vi "StateHopper.vi"(0 "Master State In":T1(ring)) -> ()   [LabVIEW 2020]
doc: "This VI makes all decisions related to the hopper subsystem."
uses:
  <vilib>/Rock Robotics/WPI/DriverStation/WPI_DriverStationAllianceInfo.ctl
  635383ba-0535-4eb4-9430-5d5cc08842cb.vi
  GlobalDriverStationCommands.vi
  GlobalHopper.vi
  GlobalDriverStationData.vi
  GlobalGripper.vi
panel:
  in  "Delay for arm clearing (ms)":u32=800
  in  "Delay for wing retraction (ms)":u32=200
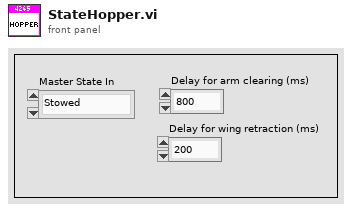
[diagram p1: front panel]
types:
  T1 = enum16{"Stowed", "Balancing", "Scoring", "Hoppering", "Ground", "Shelf"}
  T2 = typedef "WPI_DriverStationAllianceInfo.ctl" = enum16{"Red", "Blue", "Invalid"}
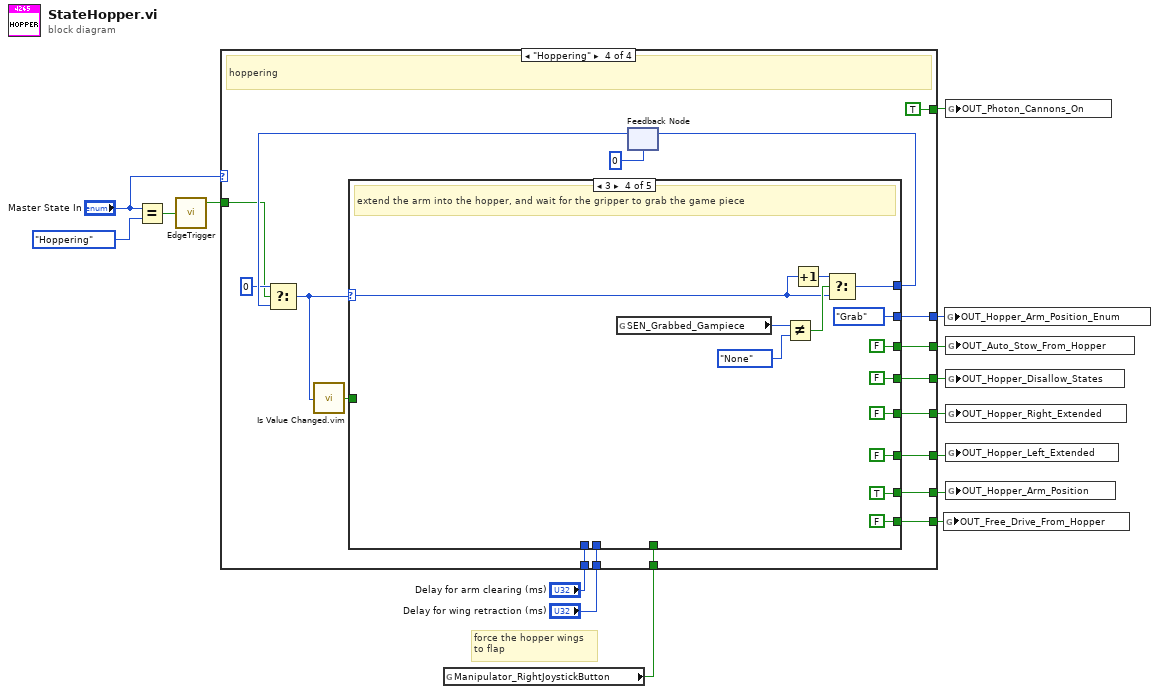
[diagram p0: block diagram]
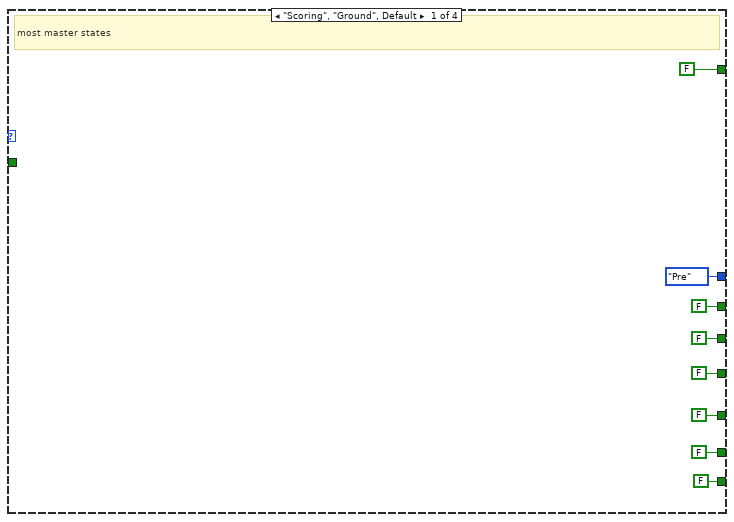
[diagram p2: hidden frame]
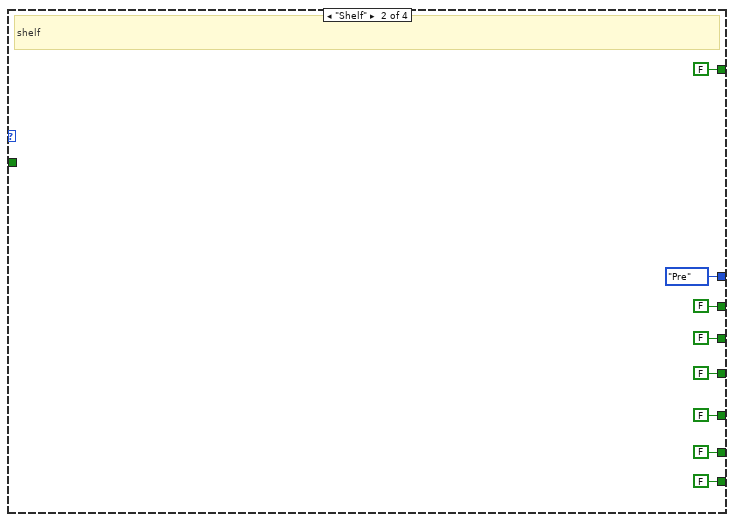
[diagram p3: hidden frame]
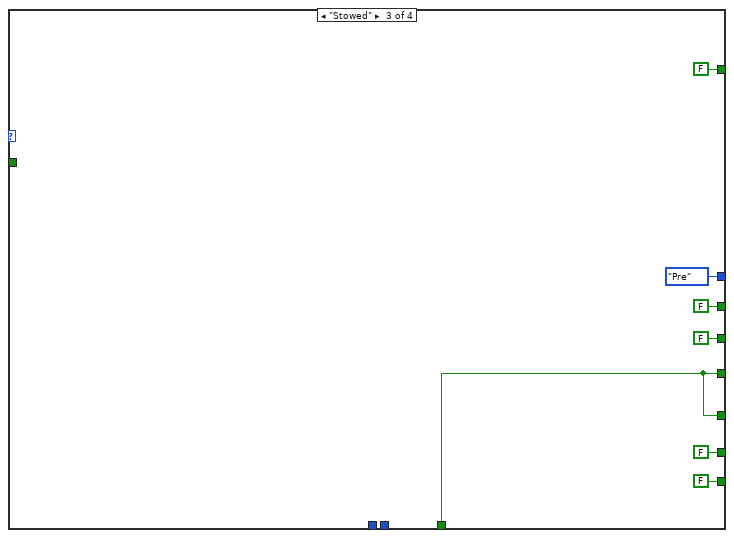
[diagram p4: hidden frame]
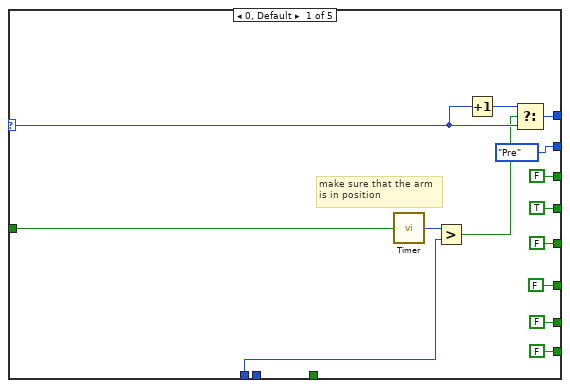
[diagram p5: hidden frame]
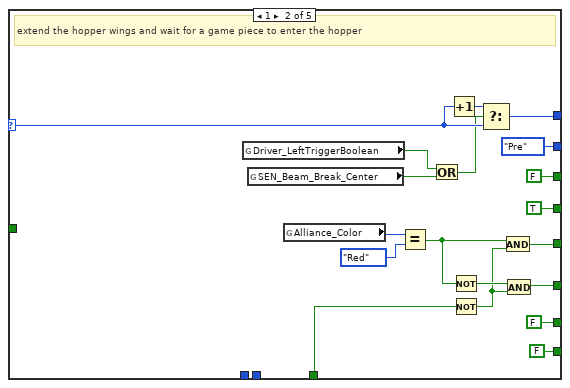
[diagram p6: hidden frame]
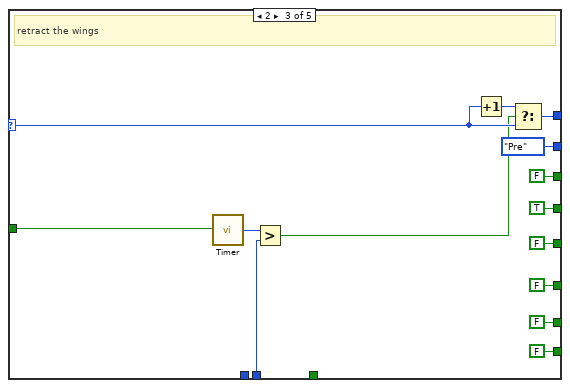
[diagram p7: hidden frame]
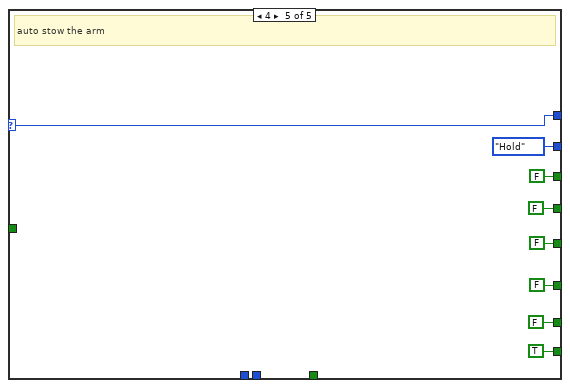
[diagram p8: hidden frame]
diagram:
  # "force the hopper wings\nto flap"
  n1 = Equal?(x="Master State In", y=T1."Hoppering") -> (x = y?=w9:bool)
  n2 = call "EdgeTrigger.vi"("Input Signal"=w9) -> ("Rising Edge Trigger"=w14:bool)  [unwired: 2 out]
  n3 = global read "GlobalDriverStationCommands.vi" "Manipulator_RightJoystickButton"() -> (w4:bool)
  n4 = case shown="\"Hoppering\"" "Master State In" {
    tunnel: w14 -> [_ _ _ w52]
    tunnel: [FALSE ("changed or first call?") FALSE ("changed or first call?") FALSE ("changed or first call?") w49] -> w13
    tunnel: [FALSE ("OUT_Hopper_Arm_Position") FALSE ("OUT_Hopper_Arm_Position") FALSE ("OUT_Hopper_Arm_Position") w48] -> w12
    tunnel: [FALSE ("OUT_Hopper_Arm_Position") FALSE ("OUT_Hopper_Arm_Position") FALSE ("OUT_Hopper_Arm_Position") w47] -> w11
    tunnel: [FALSE ("OUT_Hopper_Extended") FALSE ("New State") w35 w46] -> w10
    tunnel: "Delay for wing retraction (ms)" -> [_ _ _ w45]
    tunnel: [FALSE ("New State") FALSE ("New State") w35 w44] -> w7
    tunnel: [FALSE FALSE FALSE TRUE] -> w5
    tunnel: w4 -> [_ _ w35 w42]
    tunnel: "Delay for arm clearing (ms)" -> [_ _ _ w41]
    tunnel: [FALSE FALSE FALSE w40] -> w2
    tunnel: [enum16{"Pre", "Grab", "Hold"}."Pre" ("OUT_Hopper_Arm_Position_Enum") enum16{"Pre", "Grab", "Hold"}."Pre" ("OUT_Hopper_Arm_Position_Enum") enum16{"Pre", "Grab", "Hold"}."Pre" ("OUT_Hopper_Arm_Position_Enum") w39] -> w1
    frame "Scoring", "Ground", Default {
      # "most master states"
    }
    frame "Shelf" {
      # "shelf"
    }
    frame "Stowed" {
    }
    frame "Hoppering" {
      # "hoppering"
      n5 = feedback #1(0) -> (w54:i32)
      n6 = Select(t=0, s=w52, f=w54) -> (s? t:f=w50:i32)
      n7 = call "Is Value Changed.vim"("value"=w50) -> ("changed or first call?"=w51:bool)
      n8 = case shown="3" w50 {
        selector: w50 -> [w69 w87 w97 w113 w124]
        tunnel: [FALSE ("New State") w78 FALSE ("New State") FALSE ("Manipulator_RightJoystickButton") FALSE ("Manipulator_RightJoystickButton")] -> w46
        tunnel: [w70 w89 w99 w114 w124] -> w56
        tunnel: w51 -> [w60 _ w96 _ _]
        tunnel: [TRUE ("OUT_Hopper_Arm_Position") TRUE ("OUT_Hopper_Arm_Position") TRUE ("OUT_Hopper_Arm_Position") FALSE ("OUT_Hopper_Arm_Position") FALSE ("OUT_Hopper_Arm_Position")] -> w47
        tunnel: [FALSE ("OUT_Hopper_Arm_Position") FALSE ("OUT_Hopper_Arm_Position") FALSE ("OUT_Hopper_Arm_Position") TRUE ("OUT_Hopper_Arm_Position") FALSE ("OUT_Hopper_Arm_Position")] -> w48
        tunnel: [FALSE ("changed or first call?") FALSE ("changed or first call?") FALSE ("changed or first call?") FALSE ("changed or first call?") FALSE ("changed or first call?")] -> w49
        tunnel: w45 -> [_ _ w94 _ _]
        tunnel: [FALSE ("New State") w77 FALSE ("New State") FALSE ("Manipulator_RightJoystickButton") FALSE ("Manipulator_RightJoystickButton")] -> w44
        tunnel: w42 -> [_ w74 _ _ _]
        tunnel: w41 -> [w59 _ _ _ _]
        tunnel: [FALSE FALSE FALSE FALSE TRUE] -> w40
        tunnel: [enum16{"Pre", "Grab", "Hold"}."Pre" ("OUT_Hopper_Arm_Position_Enum") enum16{"Pre", "Grab", "Hold"}."Pre" ("OUT_Hopper_Arm_Position_Enum") enum16{"Pre", "Grab", "Hold"}."Pre" ("OUT_Hopper_Arm_Position_Enum") enum16{"Pre", "Grab", "Hold"}."Grab" ("OUT_Hopper_Arm_Position_Enum") enum16{"Pre", "Grab", "Hold"}."Hold" ("OUT_Hopper_Arm_Position_Enum")] -> w39
        frame 0, Default {
          # "make sure that the arm\nis in position"
          n9 = call "Timer.vi"("Reset Timer"=w60) -> ("Time (ms)"=w62:u32)
          n10 = Greater?(x=w62, y=w59) -> (0:w61:bool)
          n11 = Increment(x=w69) -> (x+1=w68:i32)
          n12 = Select(t=w68, s=w61, f=w69) -> (s? t:f=w70:i32)
        }
        frame 1 {
          # "extend the hopper wings and wait for a game piece to enter the hopper"
          n13 = global read "GlobalDriverStationCommands.vi" "Driver_LeftTriggerBoolean"() -> (w82:bool)
          n14 = global read "GlobalHopper.vi" "SEN_Beam_Break_Center"() -> (w81:bool)
          n15 = global read "GlobalDriverStationData.vi" "Alliance_Color"() -> (w80:T2)
          n16 = Equal?(x=w80, y=WPI_DriverStationAllianceInfo."Red") -> (x = y?=w76:bool)
          n17 = Or(x=w82, y=w81) -> (x .or. y?=w83:bool)
          n18 = Increment(x=w87) -> (x+1=w88:i32)
          n19 = Not(x=w76) -> (.not. x?=w75:bool)
          n20 = Not(x=w74) -> (.not. x?=w73:bool)
          n21 = Select(t=w88, s=w83, f=w87) -> (s? t:f=w89:i32)
          n22 = And(x=w76, y=w73) -> (x .and. y?=w78:bool)
          n23 = And(x=w75, y=w73) -> (x .and. y?=w77:bool)
        }
        frame 2 {
          # "retract the wings"
          n24 = call "Timer.vi"("Reset Timer"=w96) -> ("Time (ms)"=w95:u32)
          n25 = Greater?(x=w95, y=w94) -> (0:w93:bool)
          n26 = Increment(x=w97) -> (x+1=w98:i32)
          n27 = Select(t=w98, s=w93, f=w97) -> (s? t:f=w99:i32)
        }
        frame 3 {
          # "extend the arm into the hopper, and wait for the gripper to grab the game piece"
          n28 = global read "GlobalGripper.vi" "SEN_Grabbed_Gampiece"() -> (w108:enum16{"None", "Cube", "Cone"})
          n29 = Not Equal?(x=w108, y=enum16{"None", "Cube", "Cone"}."None") -> (x != y?=w115:bool)
          n30 = Increment(x=w113) -> (x+1=w112:i32)
          n31 = Select(t=w112, s=w115, f=w113) -> (s? t:f=w114:i32)
        }
        frame 4 {
          # "auto stow the arm"
        }
      }
      n32 = feedback-in #1(w56) -> ()
    }
  }
  n33 = global write "GlobalHopper.vi" "OUT_Free_Drive_From_Hopper"(w2) -> ()
  n34 = global write "GlobalHopper.vi" "OUT_Hopper_Arm_Position_Enum"(w1) -> ()
  n35 = global write "GlobalHopper.vi" "OUT_Photon_Cannons_On"(w5) -> ()
  n36 = global write "GlobalHopper.vi" "OUT_Auto_Stow_From_Hopper"(w13) -> ()
  n37 = global write "GlobalHopper.vi" "OUT_Hopper_Disallow_States"(w11) -> ()
  n38 = global write "GlobalHopper.vi" "OUT_Hopper_Right_Extended"(w10) -> ()
  n39 = global write "GlobalHopper.vi" "OUT_Hopper_Left_Extended"(w7) -> ()
  n40 = global write "GlobalHopper.vi" "OUT_Hopper_Arm_Position"(w12) -> ()
